vi "VI Tree.vi"   [LabVIEW 2018, in "Config.lvlib"]
uses:
  Config.lvlib
  16a0fa0a-81da-4659-b238-b71df11aec13.vi
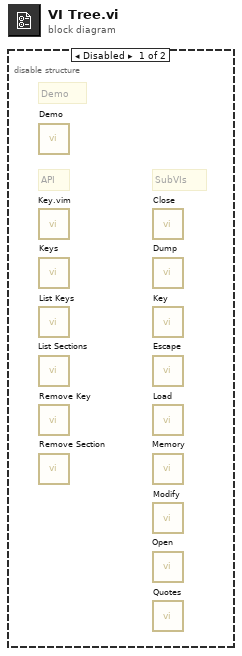
[diagram p0: block diagram]
diagram:
  n1 = disable-structure shown="Disabled" {
    frame Disabled {
      # "SubVIs"
      # "API"
      # "Demo"
      n2 = call "Demo.vi"() -> ()  [unwired: 12 in]
      n3 = call "Key.vim"() -> ()  [unwired: 8 in, 4 out]
      n4 = call "Keys.vi"() -> ()  [unwired: 9 in, 3 out]
      n5 = call "List Keys.vi"() -> ()  [unwired: 8 in, 4 out]
      n6 = call "List Sections.vi"() -> ()  [unwired: 9 in, 3 out]
      n7 = call "Remove Key.vi"() -> ()  [unwired: 9 in, 3 out]
      n8 = call "Remove Section.vi"() -> ()  [unwired: 9 in, 3 out]
      n9 = call "Close.vi"() -> ()  [unwired: 10 in, 2 out]
      n10 = call "Dump.vi"() -> ()  [unwired: 10 in, 2 out]
      n11 = call "Key.vi"() -> ()  [unwired: 8 in, 4 out]
      n12 = call "Escape.vi"() -> ()  [unwired: 10 in, 2 out]
      n13 = call "Load.vi"() -> ()  [unwired: 10 in, 2 out]
      n14 = call "Memory.vi"() -> ()  [unwired: 10 in, 2 out]
      n15 = call "Modify.vi"() -> ()  [unwired: 7 in, 5 out]
      n16 = call "Open.vi"() -> ()  [unwired: 8 in, 4 out]
      n17 = call "Quotes.vi"() -> ()  [unwired: 11 in, 1 out]
    }
    frame Enabled {
    }
  }
